vi "receive.vi"(7 "flags":i32, 8 "error in":errorcluster, 11 "socket":i64) -> (0 "error out":errorcluster, 2 "data":string)   [LabVIEW 2013, in "lvnano.lvlib"]
doc: "NN_EXPORT int nn_recv (int s, void *buf, size_t len, int flags);"
uses:
  lvnano.lvlib
  magic numbers.ctl
  lvnanomsg.dll
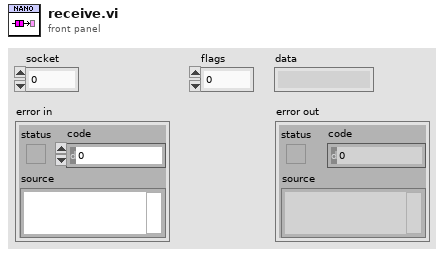
[diagram p1: front panel]
types:
  T1 = typedef "lvnano.lvlib/magic numbers.ctl" = u32
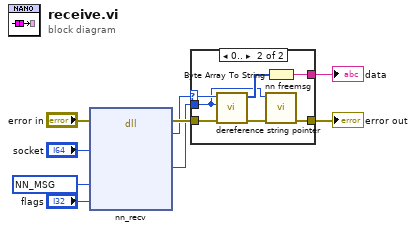
[diagram p0: block diagram]
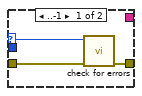
[diagram p2: hidden frame]
diagram:
  w1 = T1 4294967295 items=["NN_MSG"=4294967295] ("magic numbers")
  n1 = dll-call lib="C:/Users/Daniel/Documents/nanomsg/lvnano/lvnanomsg.*" fn="nn_recv"(error in="error in", "socket"="socket", "length"=w1, "flags"="flags") -> (error out=w6:errorcluster, "message size"=w5:i32, "data buffer"=w3:u64)  [unwired: 6 in, 1 out]
  n2 = case shown="0.." w5 {
    selector: w5 -> [w10 w18]
    tunnel: w6 -> [w11 w19]
    tunnel: [w12 w14] -> w4
    tunnel: w3 -> [_ w13]
    tunnel: [_ w17] -> w2
    frame ..-1 {
      n3 = call "check for errors.vi"("error in"=w11, "function return"=w10) -> ("error out"=w12:errorcluster)  [unwired: 9 in]
    }
    frame 0.. {
      n4 = call "dereference string pointer.vi"("error in"=w19, "data buffer"=w13, "count"=w18) -> ("error out"=w15:errorcluster, "byte array"=w16:u8[])  [unwired: 7 in]
      n5 = Byte Array To String(unsigned byte array=w16) -> (string=w17:string)
      n6 = call "nn freemsg.vi"("error in"=w15, "message pointer"=w13) -> ("error out"=w14:errorcluster)  [unwired: 9 in]
    }
  }
  "error out" <- w4
  "data" <- w2
